vi "FT_Write_String_Data.vi"(8 "error in":errorcluster, 10 "Buffer":string, 11 "Handle":u32) -> (0 "error out":errorcluster, 2 "Bytes Written":u32, 3 "Handle out":u32)   [LabVIEW 2016]
uses:
  FTD2XX.dll
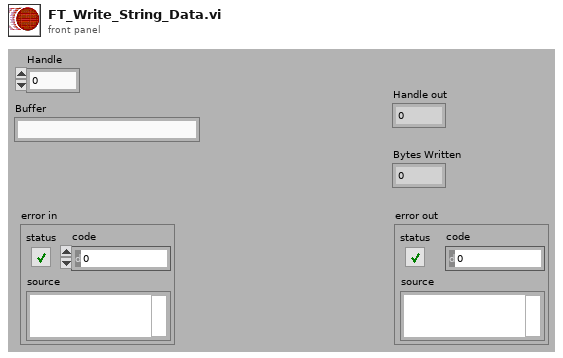
[diagram p1: front panel]
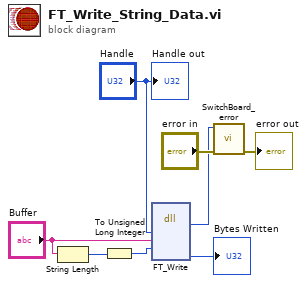
[diagram p0: block diagram]
diagram:
  n1 = String Length(string="Buffer") -> (length=w6:i32)
  n2 = To Unsigned Long Integer(number=w6) -> (unsigned 32bit integer=w5:u32)
  n3 = dll-call lib="FTD2XX.dll" fn="FT_Write"("Handle"="Handle", "Buffer"="Buffer", "BytesToWrite"=w5) -> ("FT_Status"=w2:u32, "BytesWritten"=→"Bytes Written":u32)  [unwired: 7 in, 2 out]
  n4 = call <instrlib>:"SwitchBoard_error.vi"("error constant"="error in", "Code"=w2) -> ("error IO"=→"error out":errorcluster)  [unwired: 9 in]
  "Handle out" <- "Handle"
